vi "ingresaMediciones.vi"(8 "error in (no error)":errorcluster, 10 "Selection Start":T1, 11 "Prueba09 in":refnum<class "Prueba09.lvclass">) -> (0 "error out":errorcluster, 3 "Prueba09 out":refnum<class "Prueba09.lvclass">)   [LabVIEW 2019, in "Prueba09.lvclass"]
uses:
  Prueba09.lvclass
  <vilib>/Utility/miscctls.llb/LVRowAndColumnTypeDef.ctl
  Prueba09.lvclass/Prueba09.ctl
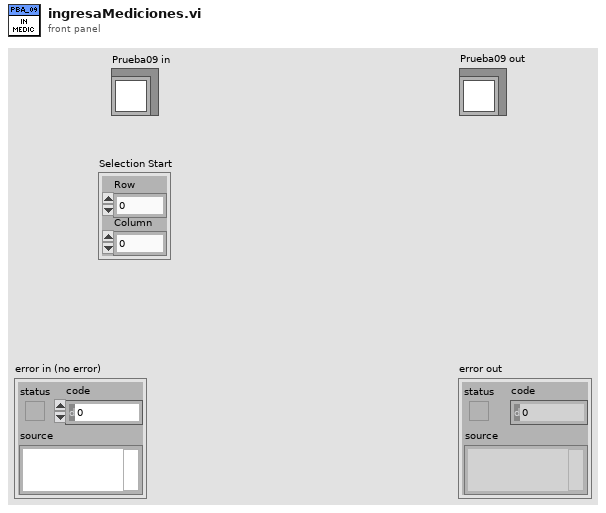
[diagram p1: front panel]
types:
  T1 = typedef "LVRowAndColumnTypeDef.ctl" = cluster{"Row":i32, "Column":i32}
  T2 = cluster{"Medido":dbl, "Error":dbl, "Ref":dbl, "Incert_exp":dbl, "Tol+":dbl, "Tol-":dbl, "fila":i32}
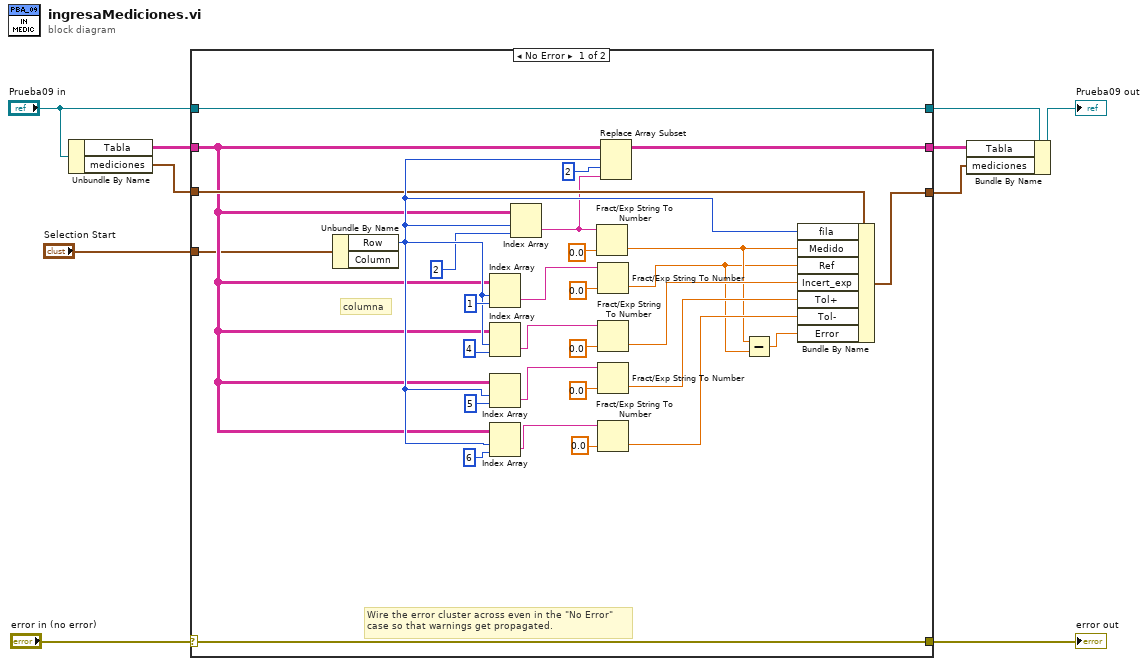
[diagram p0: block diagram]
diagram:
  n1 = Unbundle By Name("Prueba09 in") -> ("Tabla"=w6:string[][], "mediciones"=w5:T2)
  n2 = case shown="No Error" "error in (no error)" {
    selector: "error in (no error)" -> [w39 w44]
    tunnel: [w39 w44] -> w9
    tunnel: [w40 w43] -> w8
    tunnel: "Prueba09 in" -> [w40 w43]
    tunnel: w6 -> [w13 w42]
    tunnel: w5 -> [w20 w41]
    tunnel: [w19 w42] -> w3
    tunnel: [w18 w41] -> w2
    tunnel: "Selection Start" -> [w12 _]
    frame No Error {
      # "columna"
      # "Wire the error cluster across even in the \"No Error\"\ncase so that warnings get propagated."
      n3 = Unbundle By Name(w12) -> ("Row"=w21:i32)  [unwired: 1 out]
      n4 = Index Array(array=w13, index (row)=w21, index (col)=1 ("disabled index (col)")) -> (element=w35:string)
      n5 = Index Array(array=w13, index (row)=w21, index (col)=4 ("index (row)")) -> (element=w31:string)
      n6 = Index Array(array=w13, index (row)=w21, index (col)=5 ("disabled index (col)")) -> (element=w22:string)
      n7 = Index Array(array=w13, index (row)=w21, index (col)=6 ("index (row)")) -> (element=w25:string)
      n8 = Index Array(array=w13, index (row)=w21, index (col)=2 ("disabled index (col)")) -> (element=w11:string)
      n9 = Fract/Exp String To Number(string=w11, default (0 dbl)=0.0) -> (number=w17:dbl)  [unwired: 2 in, 1 out]
      n10 = Fract/Exp String To Number(string=w35, default (0 dbl)=0.0) -> (number=w16:dbl)  [unwired: 2 in, 1 out]
      n11 = Fract/Exp String To Number(string=w31, default (0 dbl)=0.0) -> (number=w30:dbl)  [unwired: 2 in, 1 out]
      n12 = Fract/Exp String To Number(string=w22, default (0 dbl)=0.0) -> (number=w23:dbl)  [unwired: 2 in, 1 out]
      n13 = Fract/Exp String To Number(string=w25, default (0 dbl)=0.0) -> (number=w24:dbl)  [unwired: 2 in, 1 out]
      n14 = Replace Array Subset(array=w13, new element=w11, index (row)=w21, index (col)=2 ("disabled index (col)")) -> (w19:string[][])
      n15 = Subtract(x=w17, y=w16) -> (x-y=w15:dbl)
      n16 = Bundle By Name(cluster=w20, "fila"=w21, "Medido"=w17, "Ref"=w16, "Incert_exp"=w30, "Tol+"=w23, "Tol-"=w24, "Error"=w15) -> (w18:T2)
    }
    frame Error {
    }
  }
  "error out" <- w9
  n17 = Bundle By Name(cluster=w8, "Tabla"=w3, "mediciones"=w2) -> (→"Prueba09 out":refnum<class "Prueba09.lvclass">)
